vi "Get IPS120 State.vi"(8 "Error In":errorcluster, 11 "VISA resource name":refnum<visa-resource-name>) -> (0 "Error Out":errorcluster, 2 "IPS state":T1, 3 "VISA resource name out":refnum<visa-resource-name>)   [LabVIEW 2018]
uses:
  IPS state.ctl
  Controls/Sweep Action.ctl
  Controls/IPS LOC-REM Status.ctl
  Controls/IPS Switch Heater Status.ctl
  Controls/IPS Mode.ctl
panel:
  out "read buffer":string
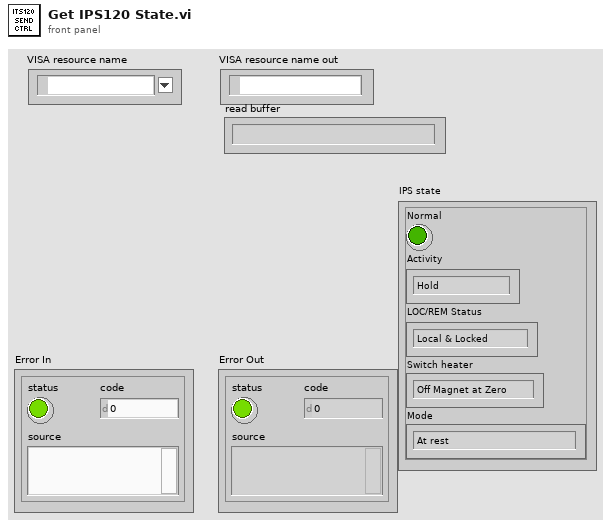
[diagram p1: front panel]
types:
  T1 = typedef "IPS state.ctl" = cluster{"Normal":bool, "Activity":T2, "LOC/REM Status":T3, "Switch heater":T4, "Mode":T5}
  T2 = typedef "Sweep Action.ctl" = enum16{"Hold", "To set point", "To zero", "Clamp"}
  T3 = typedef "IPS LOC-REM Status.ctl" = enum16{"Local & Locked", "Remote & Locked", "Local & Unlocked", "Remote & Unlocked", "Auto-Run-Down"}
  T4 = typedef "IPS Switch Heater Status.ctl" = enum16{"Off Magnet at Zero", "On", "Off Magnet at Field", "Heater Fault", "No Switch Fitted"}
  T5 = typedef "IPS Mode.ctl" = enum16{"At rest", "Sweeping", "Sweep Limiting", "Sweeping & Sweep Limiting"}
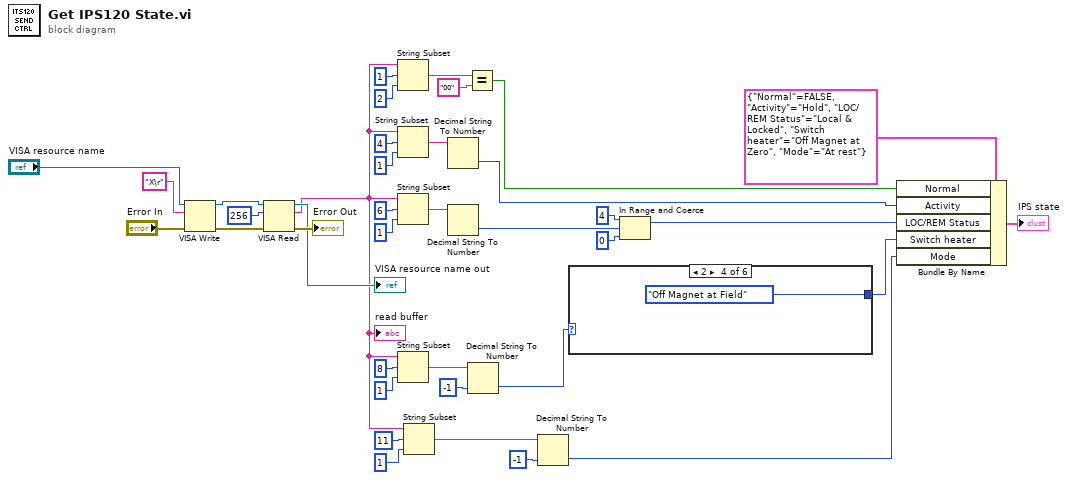
[diagram p0: block diagram]
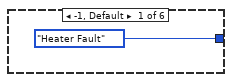
[diagram p2: hidden frame]
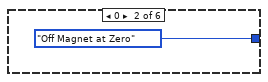
[diagram p3: hidden frame]
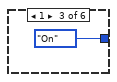
[diagram p4: hidden frame]
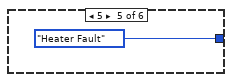
[diagram p5: hidden frame]
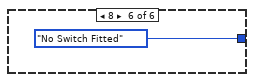
[diagram p6: hidden frame]
diagram:
  n1 = VISA Write(VISA resource name="VISA resource name", write buffer="X\r", error in (no error)="Error In") -> (VISA resource name out=w35:refnum<visa-resource-name>, error out=w37:errorcluster)  [unwired: 1 out]
  n2 = VISA Read(VISA resource name=w35, byte count=u32 256, error in (no error)=w37) -> (VISA resource name out=→"VISA resource name out":refnum<visa-resource-name>, read buffer=w3:string, error out=→"Error Out":errorcluster)  [unwired: 1 out]
  "read buffer" <- w3
  n3 = String Subset(string=w3, offset (0)=1 ("length (rest)"), length (rest)=2 ("length (rest)")) -> (substring=w26:string)
  n4 = String Subset(string=w3, offset (0)=4 ("length (rest)"), length (rest)=1 ("length (rest)")) -> (substring=w22:string)
  n5 = String Subset(string=w3, offset (0)=6 ("length (rest)"), length (rest)=1 ("length (rest)")) -> (substring=w19:string)
  n6 = String Subset(string=w3, offset (0)=8 ("length (rest)"), length (rest)=1 ("length (rest)")) -> (substring=w10:string)
  n7 = String Subset(string=w3, offset (0)=11 ("length (rest)"), length (rest)=1 ("length (rest)")) -> (substring=w6:string)
  n8 = Decimal String To Number(string=w22) -> (number=w21:i32)  [unwired: 2 in, 1 out]
  n9 = Decimal String To Number(string=w19) -> (number=w16:i32)  [unwired: 2 in, 1 out]
  n10 = Equal?(x=w26, y="00") -> (x = y?=w23:bool)
  n11 = Decimal String To Number(string=w10, default (0L)=-1 ("default (0 I32)")) -> (number=w2:i32)  [unwired: 1 in, 1 out]
  n12 = Decimal String To Number(string=w6, default (0L)=-1 ("default (0 I32)")) -> (number=w1:i32)  [unwired: 1 in, 1 out]
  n13 = case shown="2" w2 {
    tunnel: [IPS_Switch_Heater_Status."Heater Fault" ("Switch heater") IPS_Switch_Heater_Status."Off Magnet at Zero" ("Switch heater") IPS_Switch_Heater_Status."On" ("Switch heater") IPS_Switch_Heater_Status."Off Magnet at Field" ("Switch heater") IPS_Switch_Heater_Status."Heater Fault" ("Switch heater") IPS_Switch_Heater_Status."No Switch Fitted" ("Switch heater")] -> w8
    frame -1, Default {
    }
    frame 0 {
    }
    frame 1 {
    }
    frame 2 {
    }
    frame 5 {
    }
    frame 8 {
    }
  }
  n14 = In Range and Coerce(upper limit=4, x=w16, lower limit=0) -> (coerced(x)=w13:i32)  [unwired: 1 out]
  n15 = Bundle By Name(cluster=T1 {"Normal"=FALSE, "Activity"=enum."Hold", "LOC/REM Status"=enum."Local & Locked", "Switch heater"=enum."Off Magnet at Zero", "Mode"=enum."At rest"} ("IPS state"), "Normal"=w23, "Activity"=w21, "LOC/REM Status"=w13, "Switch heater"=w8, "Mode"=w1) -> (→"IPS state":T1)
